vi "Set Login Hint.vi"(10 "Login Hint":string, 11 "Request in":refnum<class "Request.lvclass">) -> (3 "Request out":refnum<class "Request.lvclass">)   [LabVIEW 2020, in "OAuth2.lvlib" / "Request.lvclass"]
uses:
  Request.lvclass
  Request.lvclass/Request.ctl
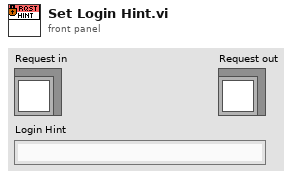
[diagram p1: front panel]
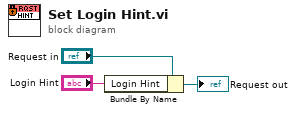
[diagram p0: block diagram]
diagram:
  n1 = Bundle By Name(cluster="Request in", "Login Hint"="Login Hint") -> (→"Request out":refnum<class "Request.lvclass">)
